vi "Get Valid Channels to Write.vi"(8 "error in (no error)":errorcluster, 9 "Data to Write In":cluster{dbl[], string[]}, 10 "Stream Names In":string[](array[string]), 11 "Plugin in":refnum<class "Sift Stream.lvclass">) -> (0 "error out":errorcluster, 1 "Data to Write Out":cluster{dbl[], string[]}, 2 "Stream Names Out":string[](array[string]), 3 "Plugin out":refnum<class "Sift Stream.lvclass">)   [LabVIEW 2024, in "Sift Stream.lvlib" / "Sift Stream.lvclass"]
uses:
  Sift Stream.lvclass
  C:/Program Files/National Instruments/LabVIEW 2024/vi.lib/FlexLogger/SDK/PluginSDK.lvlibp/PEFClasses/SDK/Plugin/Plugin.lvclass
  <vilib>/FlexLogger/SDK/PluginSDK.lvlibp/PEFClasses/SDK/Plugin/Get Valid Consumer Channels.vi
  <vilib>/FlexLogger/SDK/PluginSDK.lvlibp/PEFClasses/SDK/Consumer Channel/Consumer Channel.lvclass
  Sift Stream.lvclass/Sift Stream.ctl
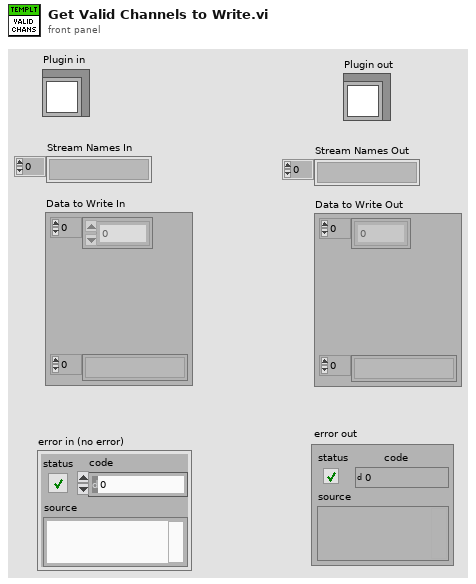
[diagram p1: front panel]
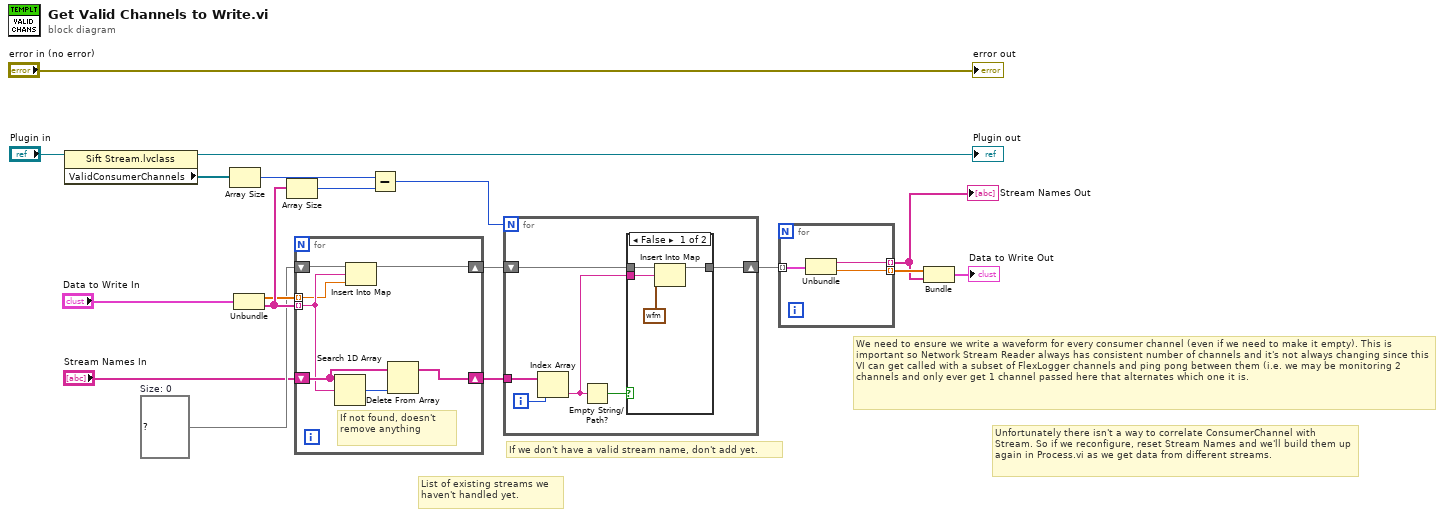
[diagram p0: block diagram]
diagram:
  w10 = map{string, dbl} {}  # Size: 0
  # "If we don't have a valid stream name, don't add yet."
  # "List of existing streams we haven't handled yet."
  # "Unfortunately there isn't a way to correlate ConsumerChannel with Stream. So if we reconfigure, reset Stream Names and we'll build them up again in Process.vi as we get data from different streams."
  # "We need to ensure we write a waveform for every consumer channel (even if we need to make it empty). This is important so Network Stream Reader always has consistent number of channels and it's not always changing since this VI can get called with a subset of FlexLogger channels and ping pong between them (i.e. we may be monitoring 2 channels and only ever get 1 channel passed here that alternates which one it is."
  n1 = property class="Sift Stream.lvclass"(reference="Plugin in") -> (reference out=→"Plugin out":refnum<class "Sift Stream.lvclass">, "ValidConsumerChannels"=w5:refnum<class "Consumer Channel.lvclass">[])  [unwired: 1 in, 1 out]
  n2 = Array Size(array=w5) -> (size(s)=w17:i32)
  n3 = Unbundle("Data to Write In") -> (w11:dbl[], w13:string[])
  n4 = Array Size(array=w13) -> (size(s)=w16:i32)
  n5 = for {
    tunnel: w13 -> [w22] mode=indexing
    shift-right: [w23] -> w14
    shift-left: "Stream Names In" -> [w25]
    tunnel: w11 -> [w21] mode=indexing
    shift-right: [w20] -> w9
    shift-left: w10 -> [w19]
    # "If not found, doesn't remove anything"
    n6 = Search 1D Array(1D array=w25, element=w22) -> (index of element=w24:i32)  [unwired: 1 in]
    n7 = Insert Into Map(map in=w19, key=w22, value=w21) -> (map out=w20:map{string, dbl})  [unwired: 2 out]
    n8 = Delete From Array(array=w25, index=w24) -> (array with subset deleted=w23:string[])  [unwired: 1 in, 1 out]
  }
  n9 = Subtract(x=w17, y=w16) -> (x-y=w15:i32)
  n10 = for {
    N: w15 -> [_]
    tunnel: w14 -> [w31]
    shift-right: [w26] -> w8
    shift-left: w9 -> [w28]
    i -> [w30]
    n11 = Index Array(array=w31, index=w30) -> (element=w27:string)
    n12 = Empty String/Path?(string/path=w27) -> (empty?=w29:bool)
    n13 = case shown="False" w29 {
      tunnel: w28 -> [w35 w36]
      tunnel: w27 -> [w34 _]
      tunnel: [w32 w36] -> w26
      frame False {
        n14 = Insert Into Map(map in=w35, key=w34, value=waveform(dbl) {"t0"=timestamp(0 s since 1904-01-01), "dt"=1.0, "Y"=[]} ("Waveform")) -> (map out=w32:map{string, dbl})  [unwired: 2 out]
      }
      frame True {
      }
    }
  }
  n15 = for {
    tunnel: w8 -> [w39] mode=indexing
    tunnel: [w38] -> w3 mode=indexing
    tunnel: [w37] -> w7 mode=indexing
    n16 = Unbundle(w39) -> (w38:string, "Waveform"=w37:dbl)
  }
  "Stream Names Out" <- w3
  n17 = Bundle(w7, w3) -> (→"Data to Write Out":cluster{dbl[], string[]})  [unwired: 1 in]
  "error out" <- "error in (no error)"
